vi "Zero-Order Hold (DBL Array).vi"(2 "initialize":bool, 3 "hold time in cycles":i32, 5 "input points":dbl[](array[numeric]) format="%.2f") -> (1 "output points":dbl[](array[numeric]) format="%.2f")   [LabVIEW 2017, in "NI_AdvCtrl_discrete linear.lvlib"]
doc: "LabVIEW no longer supports this VI. You can obtain similar functionality by installing the LabVIEW Simulation Module.\n\nHolds the signal for a definite period of time. In other words, the prediction of the signal is based only on the current value."
uses:
  <vilib>/addons/control/advanced/NI_AdvCtrl_discrete linear.lvlib
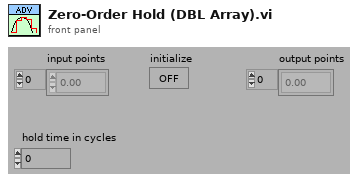
[diagram p1: front panel]
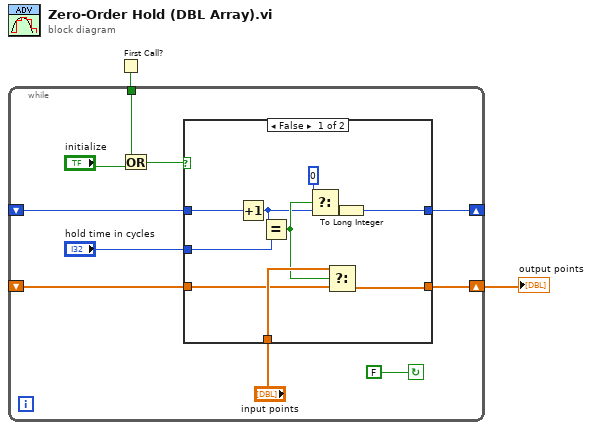
[diagram p0: block diagram]
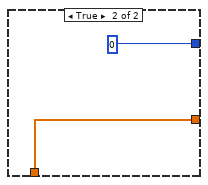
[diagram p2: hidden frame]
diagram:
  n1 = First Call?() -> (First Call?: T/F=w2:bool)
  n2 = while {
    tunnel: w2 -> [w5]
    shift-left: _ -> [w10]
    shift-right: [w11] -> _
    shift-left: _ -> [w9]
    shift-right: [w12] -> w1
    stop <- FALSE continue-if-true
    n3 = Or(x=w5, y="initialize") -> (x .or. y?=w4:bool)
    n4 = case shown="False" w4 {
      tunnel: [w17 0] -> w11
      tunnel: [w18 w24] -> w12
      tunnel: w10 -> [w22 _]
      tunnel: w9 -> [w19 _]
      tunnel: "input points" -> [w20 w24]
      tunnel: "hold time in cycles" -> [w21 _]
      frame False {
        n5 = Increment(x=w22) -> (x+1=w15:i32)
        n6 = Equal?(x=w15, y=w21) -> (x = y?=w16:bool)
        n7 = Select(t=0, s=w16, f=w15) -> (s? t:f=w13:i32)
        n8 = Select(t=w20, s=w16, f=w19) -> (s? t:f=w18:dbl[])
        n9 = To Long Integer(number=w13) -> (32bit integer=w17:i32)
      }
      frame True {
      }
    }
  }
  "output points" <- w1
